vi "Actor Core.vi"(8 "error in":errorcluster, 11 "BasicAutoRegistrationView In":refnum<class "BasicAutoRegistrationView.lvclass">) -> (0 "error out":errorcluster, 3 "Actor out":refnum<class "Actor.lvclass">)   [LabVIEW 2017, in "TestViewables.lvlib" / "BasicAutoRegistrationView.lvclass"]
doc: "(<B>Filename</B>: Actor Framework.lvlib:Actor.lvclass:Actor Core.vi)\n\nReceives messages to the actor, reacts to them, and initiates any error handling that may shut the actor down.\n\nDescendant classes may override this VI to append parallel tasks for the actor to complete while it handles messages. Overrides use the Call Parent Method node.\n\n<License>\nCopyright © 2017 Composed Systems, LLC | All rights reserved\nwww.composed.io\n\nAuthor: Ethan Stern <ethan.stern@composed.io>\n\nThis software is provided \"AS IS\" WITHOUT WARRANTIES, either express or implied, AND IS FOR EDUCATIONAL PURPOSES ONLY.\n</License>"
uses:
  BasicAutoRegistrationView.lvclass
  C:/Program Files (x86)/National Instruments/LabVIEW 2017/vi.lib/ActorFramework/Actor/Actor.lvclass
  <vilib>/ActorFramework/Actor/Actor.lvclass
  <vilib>/ActorFramework/Actor/Actor.lvclass/Actor.ctl
  <vilib>/ActorFramework/Message Enqueuer/Message Enqueuer.lvclass/Message Enqueuer.ctl
  <vilib>/ActorFramework/Message Enqueuer/Init from Existing Queue.vi
  Source/Framework/IViewable/IViewable/IViewable.lvclass
  <vilib>/ActorFramework/Message Enqueuer/Message Enqueuer.lvclass
  Source/Framework/ActorEvents/AutoRegistration/AutoRegistration.lvclass
  Source/Framework/ActorEvents/IEventAggregator Messages/ValueChangeMsg/ValueChangeMsg.lvclass
panel:
  in  "Latch When Released":bool
  in  "Latch Until Released":bool
  in  "Switch Until Released":bool
  in  "Switch When Released":bool
  in  "Latch When Pressed":bool
  in  "Switch When Pressed":bool
  # "If recursive transparency\nis broken or disabled, the\nbackground color of this\nFront Panel is red!\n(Single Pane VI)"
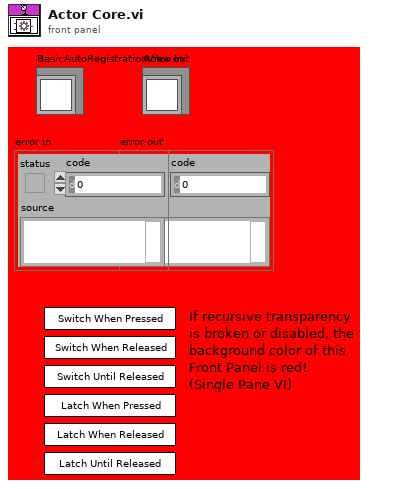
[diagram p1: front panel]
types:
  T1 = typedef "AutoRegistration.lvlib/AutoRegistration.lvclass/Auto-Event Registration Refnum.ctl" = refnum<event-registration>
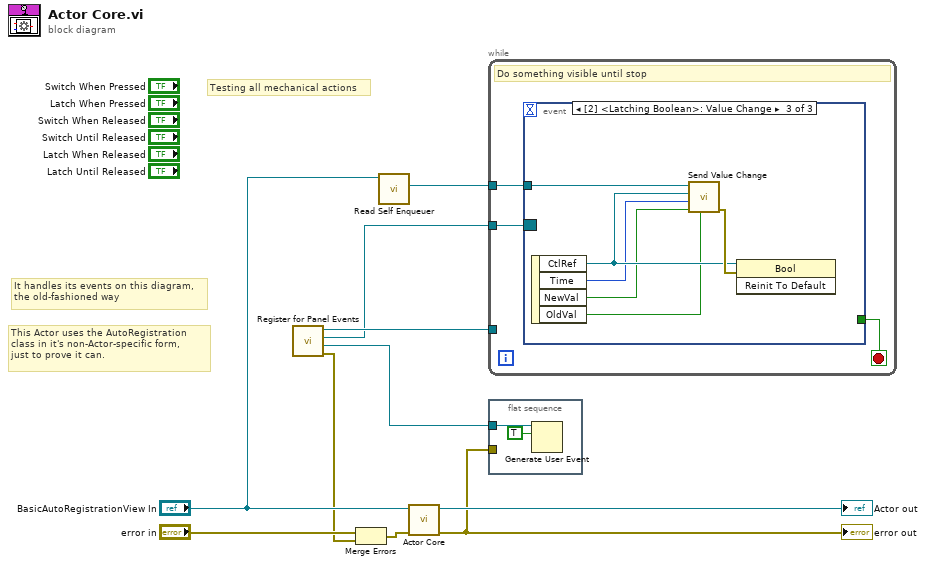
[diagram p0: block diagram]
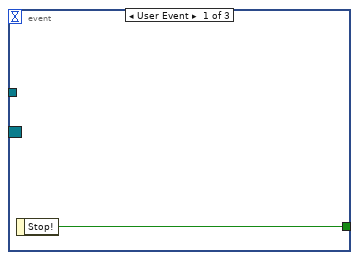
[diagram p2: hidden frame]
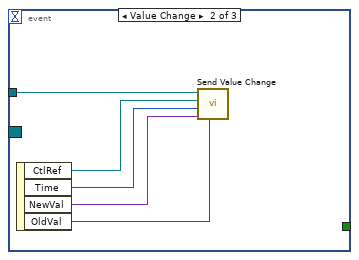
[diagram p3: hidden frame]
diagram:
  # "Testing all mechanical actions"
  # "It handles its events on this diagram,\nthe old-fashioned way"
  # "This Actor uses the AutoRegistration\nclass in it's non-Actor-specific form,\njust to prove it can."
  n1 = call "Register for Panel Events.vi"() -> ("error out"=w3:errorcluster, "Stop! Event"=w5:refnum<user-event>, "Auto-Event Registration Refnum"=w1:T1, "AbstractAutoRegistration out"=w2:refnum<class "AutoRegistration.lvclass">)  [unwired: 8 in]
  n2 = Merge Errors("error in", w3) -> (w4:errorcluster)
  n3 = call <vilib>:"Read Self Enqueuer.vi"("Actor"="BasicAutoRegistrationView In") -> ("Self Enqueuer"=w6:refnum<class "Message Enqueuer.lvclass">)  [unwired: 10 in]
  n4 = call-parent "Actor Core.vi"("error in"=w4, "IViewable In"="BasicAutoRegistrationView In") -> ("error out"=w8:errorcluster, "Actor out"=→"Actor out":refnum<class "Actor.lvclass">)  [unwired: 8 in]
  "error out" <- w8
  n5 = while {
    tunnel: w6 -> [w12]
    tunnel: w2 -> [_]
    tunnel: w1 -> [w11]
    stop <- w13 stop-if-true
    # "Do something visible until stop"
    n6 = event shown="[2] <Latching Boolean>: Value Change" {
      selector: w11 -> [_ _ _]
      dyn-events: _ -> [_ _ _]
      timeout: _ -> [_ _ _]
      tunnel: [w14 _ _] -> w13
      tunnel: w12 -> [_ w19 w25]
      event User Event {
        n7 = event-data() -> ("Stop!"=w14:bool)  [unwired: 1 in]
      }
      event Value Change {
        n8 = event-data() -> ("CtlRef"=w18:refnum<vi>, "Time"=w17:u32, "NewVal"=w16:variant, "OldVal"=w15:variant)  [unwired: 1 in]
        n9 = call "Send Value Change.vi"("Old Value"=w15, "New Value"=w16, "Time"=w17, "Ctl Refnum"=w18, "Message Enqueuer in"=w19) -> ()  [unwired: 6 in, 1 out]
      }
      event Value Change {
        n10 = event-data() -> ("CtlRef"=w23:refnum<vi>, "Time"=w22:u32, "NewVal"=w21:bool, "OldVal"=w20:bool)  [unwired: 1 in]
        n11 = call "Send Value Change.vi"("Old Value"=w20, "New Value"=w21, "Time"=w22, "Ctl Refnum"=w23, "Message Enqueuer in"=w25) -> ("error out"=w24:errorcluster)  [unwired: 6 in]
        n12 = invoke class="Bool" method="Reinit To Default"(reference=w23, error in=w24) -> ()  [unwired: 1 in, 3 out]
      }
    }
  }
  n13 = flat-sequence {
    tunnel: w5 -> [w27]
    tunnel: w8 -> [_]
    frame #0 {
      n14 = Generate User Event(user event=w27, event data cluster=TRUE ("event data")) -> ()  [unwired: 2 in, 2 out]
    }
  }
